vi "TDC_example.vi"() -> ()   [LabVIEW 2011]
panel:
  in  "Device ID":i32
  out "Exposure Time [s]":dbl
  out "Events B":i32
  out "Events A":i32
  out "Error Out":errorcluster
  out "Too Large":i32
  out "Too Small":i32
  out "Count":i32
  out "Channel Indep. Histogram":i32[](graph)
  in  "stop":bool
  in  "Selftest Period [20ns]":i32
  in  "Histogram Bin Width":i32
  in  "Histogram Bin Count":i32
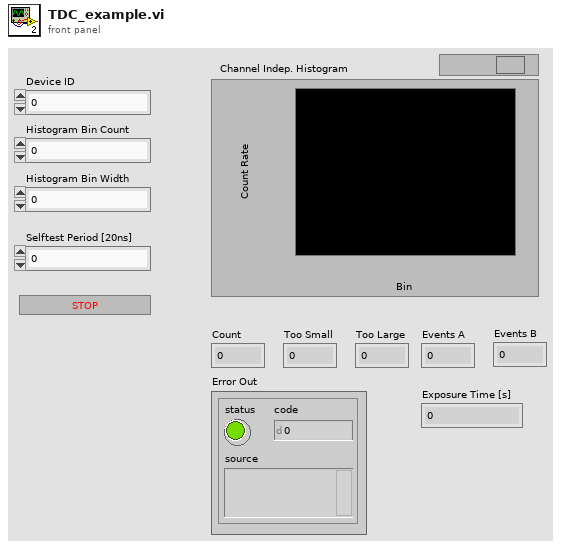
[diagram p1: front panel]
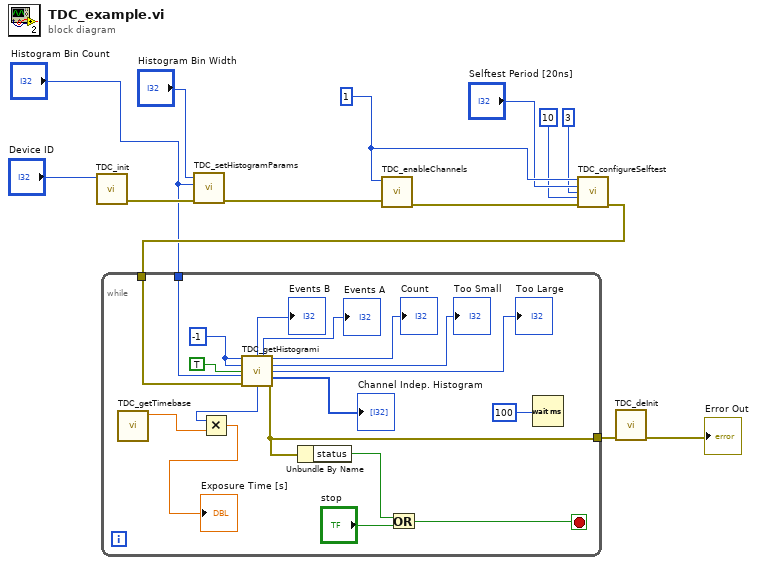
[diagram p0: block diagram]
diagram:
  w9 = 1
  n1 = call "TDC_init.vi"("Device ID"="Device ID") -> ("Error Out"=w12:errorcluster)  [unwired: 10 in]
  n2 = call "TDC_setHistogramParams.vi"("Error In"=w12, "Bin Count"="Histogram Bin Count", "Bin Width [native bins]"="Histogram Bin Width") -> ("Error Out"=w13:errorcluster)  [unwired: 8 in]
  n3 = call "TDC_enableChannels.vi"("Error In"=w13, "channelMask"=w9) -> ("Error Out"=w10:errorcluster)  [unwired: 9 in]
  n4 = call "TDC_configureSelftest.vi"("Channel Mask"=w9, "Period [20ns]"="Selftest Period [20ns]", "Burst Size"=3, "Burst Distance [80 ns]"=10, "Error In"=w10) -> ("Error Out"=w5:errorcluster)  [unwired: 10 in]
  n5 = while {
    tunnel: w5 -> [w31]
    tunnel: "Histogram Bin Count" -> [w30]
    tunnel: [w20] -> w3
    stop <- w23 stop-if-true
    w28 = -1
    n6 = call "TDC_getTimebase.vi"() -> ("Time Base [s]"=w15:dbl)  [unwired: 11 in]
    n7 = call "TDC_getHistogrami.vi"("Channel A"=w28, "Channel B"=w28, "Reset"=TRUE, "Histogram Size"=w30, "Error In"=w31) -> ("Events B"=→"Events B":i32, "Events A"=→"Events A":i32, "Data Count"=→"Count":i32, "TooSmall"=→"Too Small":i32, "TooLarge"=→"Too Large":i32, "Data"=→"Channel Indep. Histogram":i32[], "Exposure Time"=w16:i64, "Error Out"=w20:errorcluster)  [unwired: 3 in]
    n8 = Multiply(x=w16, y=w15) -> (x*y=→"Exposure Time [s]":dbl)
    n9 = Unbundle By Name(w20) -> ("status"=w22:bool)
    n10 = Or(x=w22, y="stop") -> (x .or. y?=w23:bool)
    n11 = Wait (ms)(milliseconds to wait=100) -> ()  [unwired: 1 out]
  }
  n12 = call "TDC_deInit.vi"("Error In"=w3) -> ("Error Out"=→"Error Out":errorcluster)  [unwired: 10 in]
